vi "Init Ring Acquisition.vi"(8 "error in (no error)":errorcluster, 10 "Ring Buffer Size":u32, 11 "Camera Base in":refnum<class "Camera Base.lvclass">) -> (0 "error out":errorcluster, 3 "Camera Base out":refnum<class "Camera Base.lvclass">)   [LabVIEW 2023, in "Camera Base.lvclass"]
uses:
  Camera Base.lvclass
  Camera Base.lvclass/Camera Base.ctl
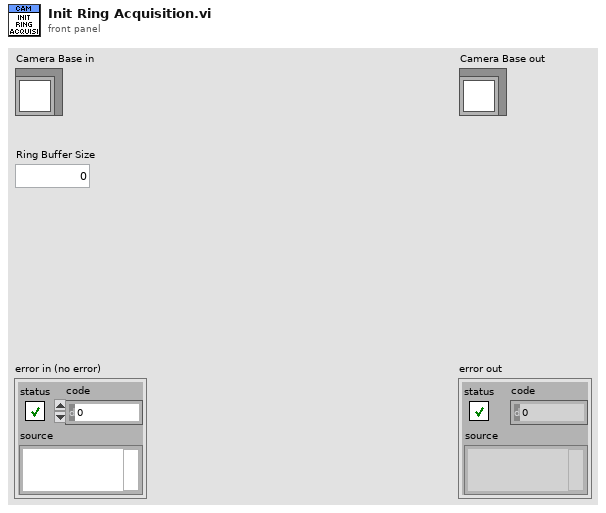
[diagram p1: front panel]
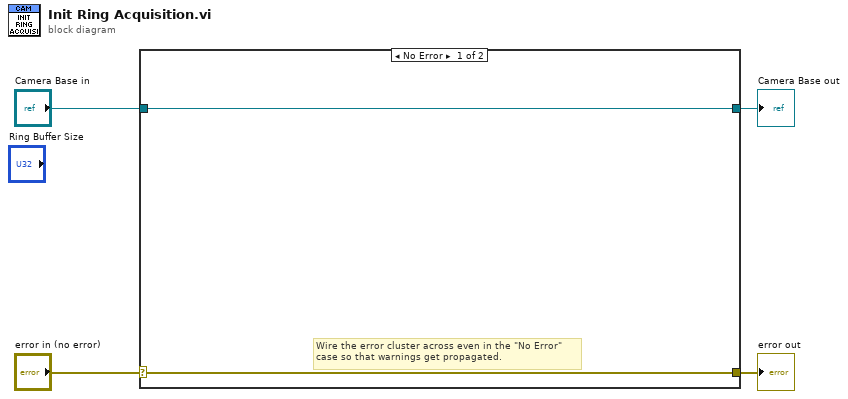
[diagram p0: block diagram]
diagram:
  n1 = case shown="No Error" "error in (no error)" {
    selector: "error in (no error)" -> [w5 w8]
    tunnel: [w5 w8] -> w3
    tunnel: [w6 w7] -> w1
    tunnel: "Camera Base in" -> [w6 w7]
    frame No Error {
      # "Wire the error cluster across even in the \"No Error\"\ncase so that warnings get propagated."
    }
    frame Error {
    }
  }
  "error out" <- w3
  "Camera Base out" <- w1
